vi "RVC 2D Homogenious Transformation.vi"() -> ()   [LabVIEW 2013]
uses:
  <vilib>/Analysis/baseanly.llb/Real A x B.vi
  <vilib>/Analysis/baseanly.llb/Real Inverse Matrix.vi
  <vilib>/Analysis/NI_AALBase.lvlib
panel:
  out "Y1":dbl=1.7320508075688776 format="%#_5g"
  out "X1":dbl=1.7320508075688776 format="%#_5g"
  in  "Y0":dbl=2.0 format="%#_13g"
  in  "X0":dbl=3.0 format="%#_13g"
  in  "stop":bool
  in  "y":dbl(slide)=2.0 scale=0.0..4.0
  in  "x":dbl(slide)=1.0 scale=0.0..4.0
  in  "angle":dbl(knob)=30.0 scale=180.0..-180.0
  out "XY Graph":cluster{dbl[], dbl[]}[](graph)=[{[1.0, 0.5, 0.49875, 0.4990849364905389, 0.5034150635094611, 0.49875, 0.4975, 0.4981698729810778, 0.5068301270189222, 0.4975, 0.49625, 0.4972548094716167, 0.5102451905283832, 0.49625, 0.495, 0.49633974596215563, 0.5136602540378444, 0.495, 0.49375, 0.4954246824526945, 0.5170753175473055, 0.49375, 0.4925, 0.4945096189432334, 0.5204903810567666, 0.4925, 0.49125, 0.49359455543377234, 0.5239054445662277, 0.49125, 0.49, 0.4926794919243112, 0.5273205080756888, 0.49, 0.48875, 0.49176442841485013, 0.5307355715851498, 0.48875, 0.4875, 0.49084936490538905, 0.5341506350946109, 0.4875, 0.48625, 0.4899343013959279, 0.5375656986040721, 0.48625, 0.485, 0.48901923788646684, 0.5409807621135332, 0.485, 0.48375, 0.4881041743770057, 0.5443958256229943, 0.48375, 0.4825, 0.48718911086754463, 0.5478108891324553, 0.4825, 0.48125, 0.48627404735808355, 0.5512259526419164, 0.48125, 0.48, 0.4853589838486224, 0.5546410161513775, 0.48, 0.47875, 0.48444392033916134, 0.5580560796608386, 0.47875, 0.47750000000000004, 0.48352885682970026, 0.5614711431702998, 0.47750000000000004, 0.47625, 0.4826137933202391, 0.5648862066797609, 0.47625, 0.47500000000000003, 0.48169872981077805, 0.5683012701892219, 0.47500000000000003, nan, 1.0, 1.8660254037844388, 1.8681904672938998, 1.8626103402749776, 1.8651103402749778, 1.8681904672938998, 1.870355530803361, 1.8591952767655167, 1.8641952767655166, 1.870355530803361, 1.872520594312822, 1.8557802132560555, 1.8632802132560555, 1.872520594312822, 1.8746856578222832, 1.8523651497465945, 1.8623651497465945, 1.8746856578222832, 1.8768507213317442, 1.8489500862371333, 1.8614500862371333, 1.8768507213317442, 1.8790157848412055, 1.8455350227276723, 1.8605350227276722, 1.8790157848412055, 1.8811808483506665, 1.8421199592182111, 1.8596199592182112, 1.8811808483506665, 1.8833459118601277, 1.83870489570875, 1.85870489570875, 1.8833459118601277, 1.8855109753695887, 1.835289832199289, 1.857789832199289, 1.8855109753695887, 1.88767603887905, 1.8318747686898278, 1.856874768689828, 1.88767603887905, 1.8898411023885109, 1.8284597051803668, 1.8559597051803667, 1.8898411023885109, 1.8920061658979719, 1.8250446416709056, 1.8550446416709057, 1.8920061658979719, 1.894171229407433, 1.8216295781614447, 1.8541295781614446, 1.894171229407433, 1.896336292916894, 1.8182145146519835, 1.8532145146519834, 1.896336292916894, 1.8985013564263553, 1.8147994511425223, 1.8522994511425224, 1.8985013564263553, 1.9006664199358163, 1.8113843876330613, 1.8513843876330613, 1.9006664199358163, 1.9028314834452775, 1.8079693241236001, 1.8504693241236, 1.9028314834452775, 1.9049965469547385, 1.8045542606141391, 1.849554260614139, 1.9049965469547385, 1.9071616104641997, 1.801139197104678, 1.848639197104678, 1.9071616104641997, 1.9093266739736607, 1.797724133595217, 1.8477241335952168, 1.9093266739736607], [2.0, 2.866025403784439, 2.8681904672939, 2.8626103402749776, 2.8651103402749776, 2.8681904672939, 2.870355530803361, 2.8591952767655164, 2.8641952767655168, 2.870355530803361, 2.8725205943128223, 2.8557802132560557, 2.8632802132560555, 2.8725205943128223, 2.8746856578222832, 2.8523651497465945, 2.8623651497465943, 2.8746856578222832, 2.8768507213317442, 2.8489500862371333, 2.8614500862371335, 2.8768507213317442, 2.8790157848412052, 2.845535022727672, 2.8605350227276722, 2.8790157848412052, 2.8811808483506667, 2.8421199592182114, 2.859619959218211, 2.8811808483506667, 2.8833459118601277, 2.83870489570875, 2.85870489570875, 2.8833459118601277, 2.8855109753695887, 2.835289832199289, 2.857789832199289, 2.8855109753695887, 2.8876760388790497, 2.831874768689828, 2.8568747686898277, 2.8876760388790497, 2.8898411023885107, 2.8284597051803666, 2.855959705180367, 2.8898411023885107, 2.892006165897972, 2.825044641670906, 2.8550446416709057, 2.892006165897972, 2.894171229407433, 2.8216295781614447, 2.8541295781614444, 2.894171229407433, 2.896336292916894, 2.8182145146519835, 2.8532145146519836, 2.896336292916894, 2.898501356426355, 2.8147994511425223, 2.8522994511425224, 2.898501356426355, 2.9006664199358165, 2.811384387633061, 2.851384387633061, 2.9006664199358165, 2.9028314834452775, 2.8079693241236003, 2.8504693241236003, 2.9028314834452775, 2.9049965469547385, 2.804554260614139, 2.849554260614139, 2.9049965469547385, 2.9071616104641995, 2.801139197104678, 2.848639197104678, 2.9071616104641995, 2.909326673973661, 2.7977241335952168, 2.847724133595217, 2.909326673973661, nan, 2.0, 2.5, 2.50125, 2.5009150635094612, 2.496584936490539, 2.50125, 2.5025, 2.501830127018922, 2.4931698729810776, 2.5025, 2.50375, 2.5027451905283833, 2.489754809471617, 2.50375, 2.505, 2.5036602540378445, 2.4863397459621557, 2.505, 2.50625, 2.5045753175473053, 2.4829246824526945, 2.50625, 2.5075, 2.5054903810567666, 2.4795096189432333, 2.5075, 2.50875, 2.506405444566228, 2.4760945554337725, 2.50875, 2.51, 2.5073205080756886, 2.4726794919243114, 2.51, 2.51125, 2.50823557158515, 2.46926442841485, 2.51125, 2.5125, 2.509150635094611, 2.465849364905389, 2.5125, 2.51375, 2.510065698604072, 2.462434301395928, 2.51375, 2.515, 2.510980762113533, 2.459019237886467, 2.515, 2.51625, 2.5118958256229944, 2.455604174377006, 2.51625, 2.5175, 2.512810889132455, 2.4521891108675447, 2.5175, 2.51875, 2.5137259526419165, 2.4487740473580835, 2.51875, 2.52, 2.5146410161513777, 2.4453589838486223, 2.52, 2.52125, 2.5155560796608385, 2.4419439203391615, 2.52125, 2.5225, 2.5164711431702997, 2.4385288568297003, 2.5225, 2.52375, 2.517386206679761, 2.435113793320239, 2.52375, 2.525, 2.518301270189222, 2.431698729810778, 2.525]}, {[3.0], [2.0]}]
  out "matrix transformation":picture
  # "Coodinate Reference System"
  # "Reference System"
  # "New Reference System"
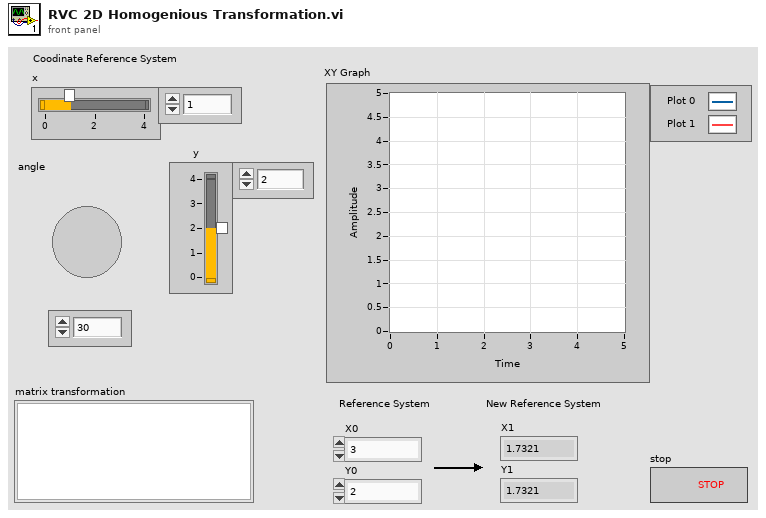
[diagram p1: front panel]
types:
  T1 = typedef "NI_Matrix.lvlib/RealMatrix.ctl" = dbl[][]
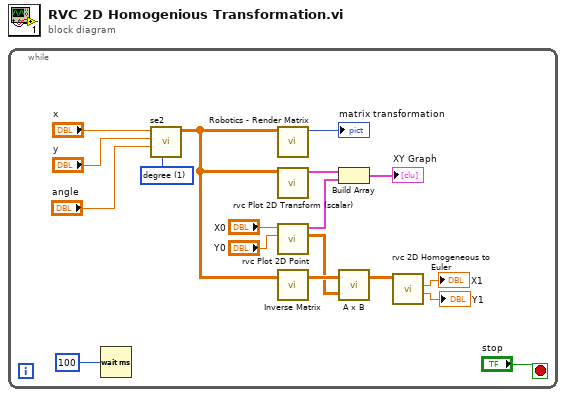
[diagram p0: block diagram]
diagram:
  n1 = while {
    stop <- "stop" stop-if-true
    w15 = u16 1 items=["radians", "degree"] ("angle unit")
    n2 = Wait (ms)(milliseconds to wait=u32 100) -> ()  [unwired: 1 out]
    n3 = call "se2.vi"("angle unit"=w15, "theta"="angle", "y"="y", "x"="x") -> ("T"=w5:dbl[][])  [unwired: 6 in, 1 out]
    n4 = call "Robotics - Render Matrix.vi"("A"=w5) -> ("picture out"=→"matrix transformation":picture)  [unwired: 10 in]
    n5 = call "rvc Plot 2D Transform (scalar).vi"("T"=w5) -> ("XY Graph 2"=w13:cluster{dbl[], dbl[]})  [unwired: 9 in, 1 out]
    n6 = call "rvc Plot 2D Point.vi"("Y"="Y0", "X"="X0") -> ("Column vector"=w4:dbl[][], "XY Graph"=w7:cluster{dbl[], dbl[]})  [unwired: 8 in]
    n7 = call-poly <vilib>:"Inverse Matrix.vi"("Input Matrix"=w5) -> ("Inverse Matrix"=w6:T1)  [unwired: 1 in, 1 out]
    n8 = Build Array(w13, w7) -> (→"XY Graph":cluster{dbl[], dbl[]}[])
    n9 = call-poly <vilib>:"A x B.vi"("B"=w4, "A"=w6) -> ("A x B"=w3:T1)  [unwired: 1 out]
    n10 = call "rvc 2D Homogeneous to Euler.vi"("T"=w3) -> ("y"=→"Y1":dbl, "x"=→"X1":dbl)  [unwired: 7 in, 2 out]
  }
